vi "CRYProject Editor PIC Set TS ListBox.vi"(10 "pRefTSListBox":refnum<vi>) -> (3 "TS Name Out":string)   [LabVIEW 2013]
uses:
  CRYProject Editor Global.vi
panel:
  in  "TS Name":u16(ring) items=["New Task Sequence"]
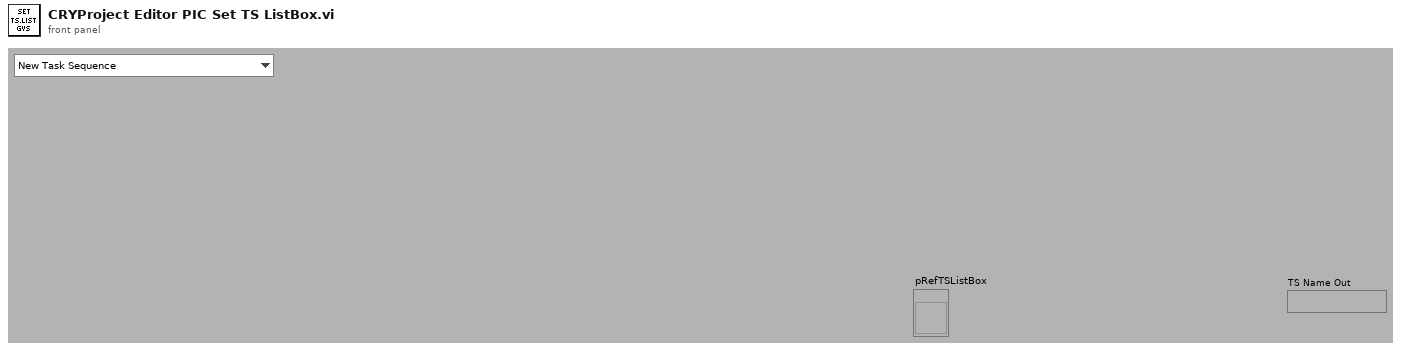
[diagram p1: front panel]
types:
  T1 = typedef "CRYTS.ctl" = cluster{"No.TS":u16, "TS File Path":path, "TS Name":string, "EditStepName":string, "Steps":T2[], "New State":bool, "Change State":bool, "Flattened CurveLib Data":string, "Document Data":string, "EditStepNo":u16, "Operator Start File":string, "Sequence Type":string, "Sequence Language":string}
  T2 = typedef "CRYStep.ctl" = cluster{"No.VI":i32, "Category":string, "StepName":string, "Seq setup flattened":string, "Comment":string, "Steps config.":bool[], "Jump config":i32[], "Start":dbl, "Increment":dbl, "Name":string, "Unit":string, "Y data":u16, "Y prefix":string, "Y dB ref":dbl, "Y unit":string, "Repeat State Array":cluster{"Start":dbl, "Increment":dbl, "Count":i32, "Num":i32}[]}
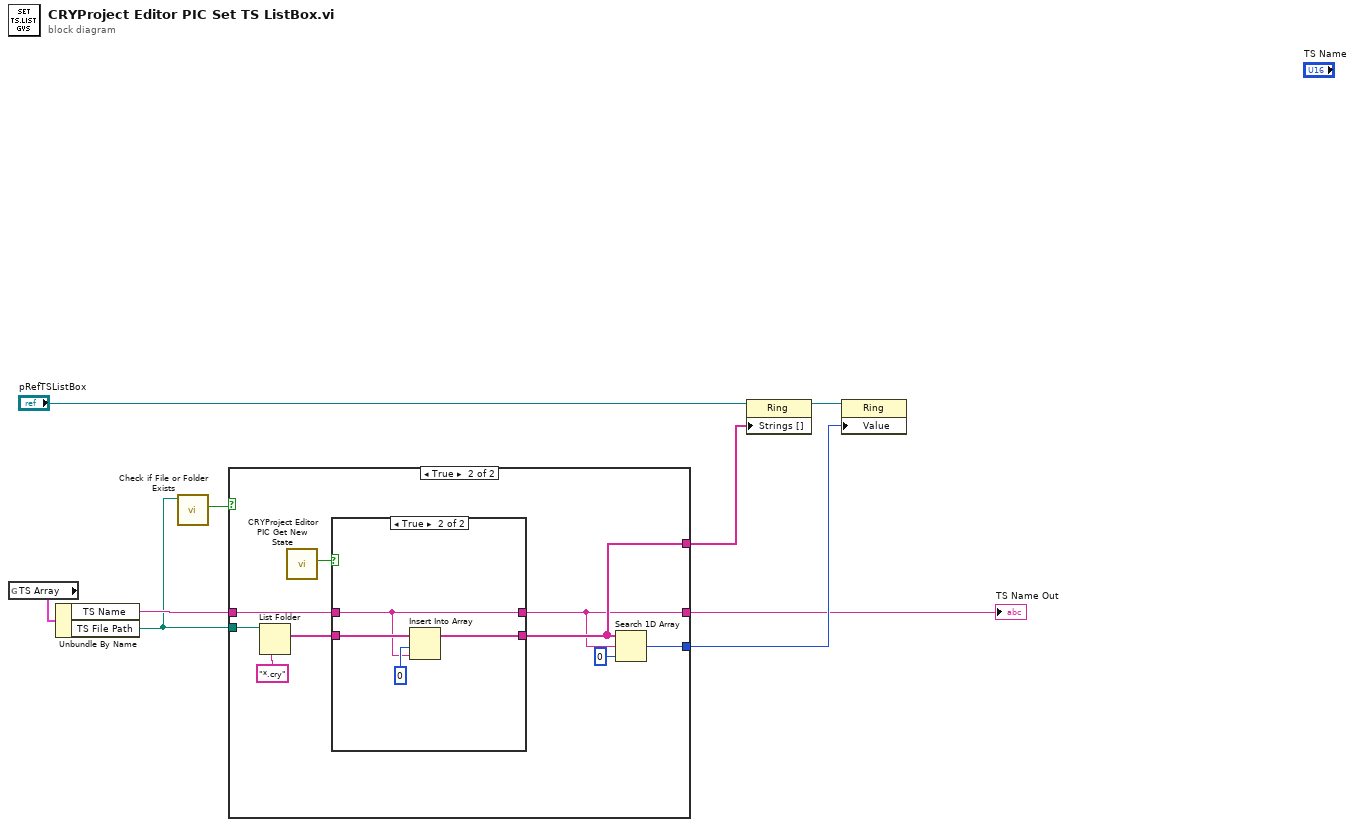
[diagram p0: block diagram]
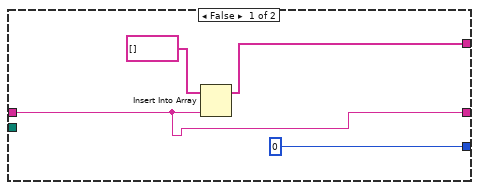
[diagram p2: hidden frame]
diagram:
  n1 = global read "CRYProject Editor Global.vi" "TS Array"() -> (w9:T1)
  n2 = Unbundle By Name(w9) -> ("TS Name"=w6:string, "TS File Path"=w3:path)
  n3 = call <vilib>:"Check if File or Folder Exists.vi"("path"=w3) -> ("file or folder exists?"=w2:bool)  [unwired: 8 in, 2 out]
  n4 = case shown="True" w2 {
    tunnel: w6 -> [w10 w17]
    tunnel: [w13 w16] -> w5
    tunnel: w3 -> [_ w22]
    tunnel: [0 ("index of element") w21] -> w4
    tunnel: [w10 w14] -> w1
    frame False {
      n5 = Insert Into Array(array=string[] [] ("Strings []"), new element=w10) -> (w13:string[])  [unwired: 1 in]
    }
    frame True {
      n6 = List Folder(path=w22, pattern="*.cry") -> (filenames=w18:string[])  [unwired: 2 in, 3 out]
      n7 = call "CRYProject Editor PIC Get New State.vi"() -> ("bNewState"=w19:bool)  [unwired: 11 in]
      n8 = case shown="True" w19 {
        tunnel: w18 -> [w23 w28]
        tunnel: w17 -> [w24 w25]
        tunnel: [w24 w25] -> w14
        tunnel: [w23 w27] -> w16
        frame False {
        }
        frame True {
          n9 = Insert Into Array(array=w28, index=0, new element=w25) -> (w27:string[])
        }
      }
      n10 = Search 1D Array(1D array=w16, element=w14, start index (0)=0) -> (index of element=w21:i32)
    }
  }
  "TS Name Out" <- w1
  n11 = property class="Ring"(reference="pRefTSListBox", "Strings []"=w5) -> (reference out=w7:refnum<vi>)  [unwired: 1 in, 1 out]
  n12 = property class="Ring"(reference=w7, "Value"=w4) -> ()  [unwired: 1 in, 2 out]
